vi "UIDatabaseAdapter.vi"(8 "error in (no error)":errorcluster, 10 "UI Data":variant, 11 "Model.lvclass":refnum<class "Model.lvclass">) -> (0 "error out":errorcluster, 2 "Database Data":variant, 3 "Model.lvclass out":refnum<class "Model.lvclass">)   [LabVIEW 2015, in "UserManagement.lvlib" / "Model.lvclass"]
uses:
  UserManagement/Model/Model.lvclass
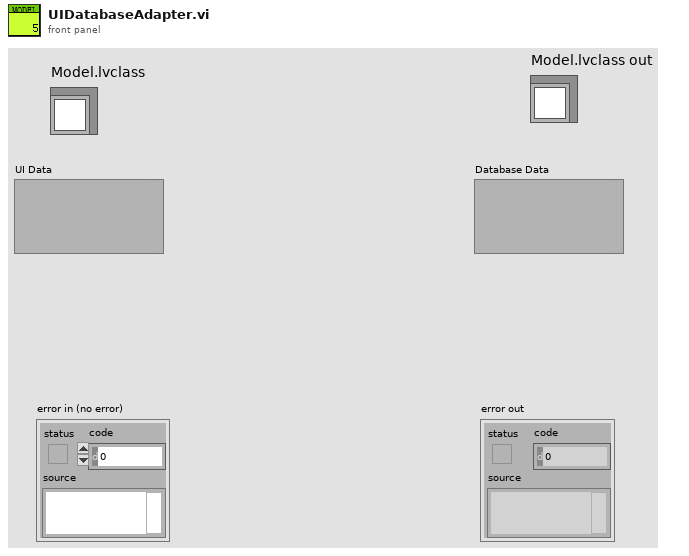
[diagram p1: front panel]
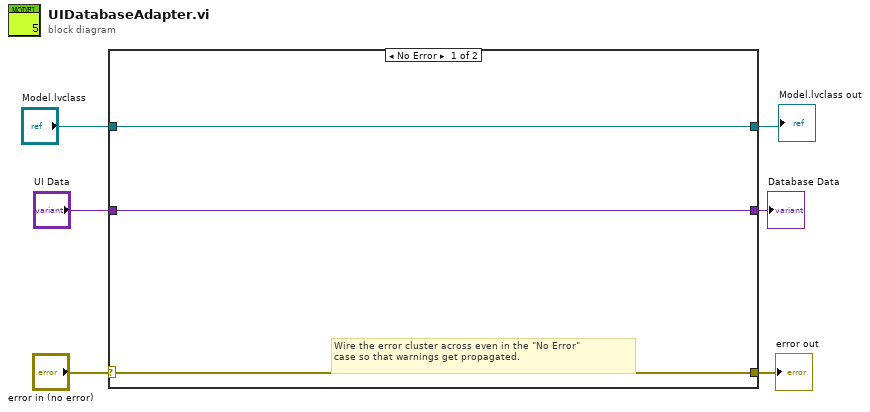
[diagram p0: block diagram]
diagram:
  n1 = case shown="No Error" "error in (no error)" {
    selector: "error in (no error)" -> [w9 w11]
    tunnel: [w9 w11] -> w5
    tunnel: "UI Data" -> [w8 _]
    tunnel: [w8 _] -> w3
    tunnel: "Model.lvclass" -> [w7 w10]
    tunnel: [w7 w10] -> w1
    frame No Error {
      # "Wire the error cluster across even in the \"No Error\"\ncase so that warnings get propagated."
    }
    frame Error {
    }
  }
  "error out" <- w5
  "Database Data" <- w3
  "Model.lvclass out" <- w1
